vi "gds_simulator.vi"() -> ()   [LabVIEW 2012]
uses:
  <vilib>/addons/Modulation/Analog/controls/Complex Data Waveform.ctl
  <vilib>/addons/Modulation/niAMT.lvlib
panel:
  in  "RX Parameters":T1={"Sampling Rate"=4000000.0, "RX Oversample Factor"=4} {"Sampling Rate" format="%^.2e"}
  in  "Shared Parameters":T2={"Packet Length"=100, "Preamble Length"=20, "modulation type"=enum."OOK", "FSK deviation (Hz)"=150000.0, "Filter Parameters"={"modulation type"=enum."ASK", "pulse shaping filter (none)"=enum."none", "filter length (symbols)"=8, "filter parameter"=0.5}} {"Filter Parameters"."filter parameter" format="%.2f"; "FSK deviation (Hz)" format="%.2p"}
  out "Measurements":T3 caption="measurements" {"FSK error (Hz)" format="%.2f"; "deviation error (Hz)" format="%.2f"; "frequency drift (Hz)" format="%.2f"; "frequency offset (Hz)" format="%.2f"}
  out "recovered complex waveform":T4={"t0"=0.0, "dt"=6.25e-08, "Y"=[1.000128536665126+0.0i, 0.751586197118696+0.0i, 0.4998027919805991+0.0i, 0.250727982644391+0.0i, -0.00043487880682959964+0.0i, 0.2509497723379846+0.0i, 0.5004826812037222+0.0i, 0.7513401422859647+0.0i, 1.0011385612332764+0.0i, 0.7507480417630159+0.0i, 0.5005377871325838+0.0i, 0.2501383829137712+0.0i, 9.932713849573499e-05+0.0i, 0.2506331619076792+0.0i, 0.5007823017747152+0.0i, 0.7512111584953517+0.0i, 1.001234869577084+0.0i, 0.7507086660409406+0.0i, 0.5005559492379272+0.0i, 0.2501286476641118+0.0i, 0.00010432492947821529+0.0i, 0.2506307378836997+0.0i, 0.5007833967235412+0.0i, 0.7512107089735025+0.0i, 1.0012350317081362+0.0i, 0.7507086187539144+0.0i, 0.5005559599140732+0.0i, 0.2501286476641118+0.0i, 0.00010432492947821529+0.0i, 0.2506307378836997+0.0i, 0.5007833967235412+0.0i, 0.7512107089735025+0.0i, 1.0012350317081362+0.0i, 0.7507086187539144+0.0i, 0.5005559599140732+0.0i, 0.2501286476641118+0.0i, 0.00010432492947821529+0.0i, 0.2506307378836997+0.0i, 0.5007833967235412+0.0i, 0.7512107089735025+0.0i, 1.0012350317081362+0.0i, 0.7507086187539144+0.0i, 0.5005559599140732+0.0i, 0.2501286476641118+0.0i, 0.00010431423258635818+0.0i, 0.25063078524390886+0.0i, 0.5007832236720497+0.0i, 0.751211206406983+0.0i, 1.0012337838864194+0.0i, 0.7507114479511843+0.0i, 0.5005500450136401+0.0i, 0.25014027313937504+0.0i, 8.257686503592398e-05+0.0i, 0.2506699648285502+0.0i, 0.5007141646378572+0.0i, 0.7513334715067744+0.0i, 1.0009882953333455+0.0i, 0.751007662665835+0.0i, 0.5000017970341639+0.0i, 0.2506829533097328+0.0i, -0.0006056489582923521+0.0i, 0.2513390899485713+0.0i, 0.5002702293185063+0.0i, 0.7516085932252198+0.0i, 1.001317612226754+0.0i, 0.7502187599744155+0.0i, 0.5016154889194743+0.0i, 0.24853596070855516+0.0i, 0.0021738712548351516+0.0i, -0.0023391492054576648+0.0i, 0.002800740735483542+0.0i, -0.0025125144170003496+0.0i, 0.0025002679488030075+0.0i, 0.24875267224128303+0.0i, 0.502021464333328+0.0i, 0.7507211811248449+0.0i, 1.0011583479909132+0.0i, 1.00220487833868+0.0i, 0.9999033167533267+0.0i, 1.003155986548728+0.0i, 0.9991551723685784+0.0i, 1.0034766480326627+0.0i, 0.9989246775240931+0.0i, 1.0034343879039176+0.0i, 0.9990847189746185+0.0i, 1.0032604247248458+0.0i, 0.9994047431658972+0.0i, 1.002969462571593+0.0i, 0.9998314632099634+0.0i, 1.002477135847846+0.0i, 1.0003820743630871+0.0i, 1.0018633881693497+0.0i, 1.0009184881961803+0.0i, 0.7507665394691232+0.0i, 0.5006961121670002+0.0i, 0.24988702932257933+0.0i, 0.0003055397879960537+0.0i, 0.25045279064926845+0.0i, 0.5008598268147144+0.0i, 0.7512071510453188+0.0i, 1.0013382778946756+0.0i, 0.7505707278325852+0.0i, 0.5011013471120391+0.0i, 0.24929199517568223+0.0i, 0.0015231595958228514+0.0i, -0.0018697074439847532+0.0i, 0.0027112989756689007+0.0i, -0.0029122396150171115+0.0i, 0.0034003770436542204+0.0i, -0.003280540022698962+0.0i, 0.0032442710783317703+0.0i, -0.002660712780105675+0.0i, 0.0022979706937644286+0.0i, 0.2493218142787346+0.0i, 0.5013616603490355+0.0i, 0.7516035360534278+0.0i, 1.0001576644674623+0.0i, 1.0031112075731934+0.0i, 0.9987144979671289+0.0i, 1.004146722051281+0.0i, 0.9979277314279233+0.0i, 1.0046493566037573+0.0i, 0.9977125025638586+0.0i, 1.00456120393046+0.0i, 0.9981645620498365+0.0i, 1.0038346518801036+0.0i, 0.9993092785373742+0.0i, 1.0024797949898978+0.0i, 1.000977081790544+0.0i, 0.7501153376048973+0.0i, 0.5022282822062422+0.0i, 0.2477947265761407+0.0i, 0.003037807810337781+0.0i, -0.0031683564583393406+0.0i, 0.0033028481784962795+0.0i, -0.002764074700312304+0.0i, 0.0022269056021686183+0.0i, 0.24948848254532183+0.0i, 0.5008020006605832+0.0i, 0.7523023342756078+0.0i, 0.9992556274212987+0.0i, 1.004070814828902+0.0i, 0.9980292197466102+0.0i, 1.0045577684621514+0.0i, 0.9981298873906143+0.0i, 0.7531425834272562+0.0i, 0.498758723598838+0.0i, 0.25092847185712436+0.0i, -8.720643290498419e-05+0.0i, -0.0007035824731183089+0.0i, 0.0012974559681197394+0.0i, -0.0016541739776803268+0.0i, 0.0019144379726028931+0.0i, -0.0018236610274930329+0.0i, 0.0018481729222402153+0.0i, -0.0015247815861743777+0.0i, 0.0015178830543329+0.0i, -0.0011643152359881285+0.0i, 0.001333604266534931+0.0i, -0.0010725457022508302+0.0i, 0.0012734272337872686+0.0i, -0.0011993122929242345+0.0i, 0.001230254232285946+0.0i, -0.0011446387399175772+0.0i, 0.0009456776883348441+0.0i, -0.0006173716355468945+0.0i, 0.0001713033320193535+0.0i, 0.00035419013214571315+0.0i, -0.0008745850549463164+0.0i, 0.2520177269110101+0.0i, 0.49878953607777865+0.0i, 0.7533668501633469+0.0i, 0.9988846730300079+0.0i, 0.7528403690283272+0.0i, 0.4986174953520837+0.0i, 0.25141652289930166+0.0i, -0.0007302000338936521+0.0i, 1.8445209841694958e-05+0.0i, 0.0008521844813141006+0.0i, -0.001426765919450218+0.0i, 0.0021852452925184536+0.0i, -0.002528438837859647+0.0i, 0.002997879955148735+0.0i, -0.0029733308332217296+0.0i, 0.00315082717819+0.0i, -0.002686677203146186+0.0i, 0.0025721301595158634+0.0i, -0.0017725634728387057+0.0i, 0.0012947516375175863+0.0i, 0.25022918449120357+0.0i, 0.5001723228969468+0.0i, 0.7525948635635091+0.0i, 0.998928932959013+0.0i, 1.004286840061977+0.0i, 0.9974960620034783+0.0i, 1.0052861584200483+0.0i, 0.996983320098374+0.0i, 1.0052685164586146+0.0i, 0.997535802997294+0.0i, 1.0042180472660442+0.0i, 0.999018700305025+0.0i, 0.7518531806360466+0.0i, 0.5004569444288187+0.0i, 0.2492225895841184+0.0i, 0.0018712067029053039+0.0i, -0.0024738914890061643+0.0i, 0.003144292967198615+0.0i, -0.003227119370524421+0.0i, 0.0033750699927966995+0.0i, -0.0029067753001163275+0.0i, 0.0027240533397893457+0.0i, -0.0019115042765191893+0.0i, 0.001668999300507921+0.0i, 0.24974726959814494+0.0i, 0.5013532809643555+0.0i, 0.7510568970786982+0.0i, 1.0013505124478064+0.0i, 0.750694697032428+0.0i, 0.5006422807187524+0.0i, 0.24994025418320215+0.0i, 0.0003180831497285305+0.0i, 0.25037272173274683+0.0i, 0.5009492404030507+0.0i, 0.7512198666659388+0.0i, 1.0010681938167683+0.0i, 1.0018149964616638+0.0i, 1.0004066247126289+0.0i, 1.0024626621963892+0.0i, 0.9998401406350473+0.0i, 1.0029656343411324+0.0i, 0.9994027843429939+0.0i, 1.0032701050433652+0.0i, 0.9990626908536583+0.0i, 1.0034760306587285+0.0i, 0.9988505269792963+0.0i, 1.003607334783805+0.0i, 0.9988964615628683+0.0i, 1.003473011367319+0.0i, 0.999320307231625+0.0i, 1.0028137466748466+0.0i, 1.000289813496653+0.0i, 0.7509903364207922+0.0i, 0.5012302976192266+0.0i, 0.2487169225826871+0.0i, 0.002410405623408453+0.0i, -0.00291987165725027+0.0i, 0.003779971804916688+0.0i, -0.0038268655079649184+0.0i, 0.004110535871290194+0.0i, -0.003630565357746327+0.0i, 0.003249390516118569+0.0i, -0.002323934836355721+0.0i, 0.0016094346023591741+0.0i, 0.25019740462392726+0.0i, 0.5003631568518416+0.0i, 0.7525267742139664+0.0i, 0.9995277131733875+0.0i, 1.0033655402096595+0.0i, 0.9991790995867168+0.0i, 1.003109171928079+0.0i, 0.9997628421906146+0.0i, 0.7516202214600886+0.0i, 0.49999724949181384+0.0i, 0.2502284540865264+0.0i, -6.589272606641215e-05+0.0i, 0.25072496167122876+0.0i, 0.5002393515812941+0.0i, 0.7520858257592368+0.0i, 0.999896445421567+0.0i, 1.0030833798673002+0.0i, 0.9991670166932658+0.0i, 1.0034188121769922+0.0i, 0.9993540508400994+0.0i, 0.7521256538962483+0.0i, 0.5000108121518518+0.0i, 0.24990091650022914+0.0i, 0.0011619766526191919+0.0i, -0.001890333330762509+0.0i, 0.0025216283810360314+0.0i, -0.0027963893182235034+0.0i, 0.0028600957266303587+0.0i, -0.002443365051434658+0.0i, 0.0020252183474949803+0.0i, -0.0011821696422666657+0.0i, 0.0006650353876859234+0.0i, 0.25081418473018074+0.0i, 0.5001923724300027+0.0i, 0.7521715419278338+0.0i, 1.000404836638586+0.0i, 0.7513420128234725+0.0i, 0.5004019124642737+0.0i, 0.24971757851375342+0.0i, 0.0009254515422090878+0.0i, -0.0013072784905761145+0.0i, 0.0015366552183685134+0.0i, -0.0014704600390226075+0.0i, 0.0012280797189567999+0.0i, 0.24997914685265876+0.0i, 0.5007278870275318+0.0i, 0.7519862062856911+0.0i, 0.9999659431859507+0.0i, 1.003123626274542+0.0i, 0.9991721084481632+0.0i, 1.0033676802504412+0.0i, 0.9992980675412391+0.0i, 0.752206405410947+0.0i, 0.4995530880585731+0.0i, 0.2505871896585888+0.0i, 3.840712565549651e-05+0.0i, 0.2502234877139924+0.0i, 0.5013047898431594+0.0i, 0.7504903125448779+0.0i, 1.0019672595444384+0.0i, 0.7501129012488448+0.0i, 0.5011848796153869+0.0i, 0.24969454663249652+0.0i, 0.0006218040972395145+0.0i, 0.25016400162887775+0.0i, 0.5014883194234692+0.0i, 0.7504697015769647+0.0i, 1.0022607543615492+0.0i, 0.749602476677032+0.0i, 0.5017861005341123+0.0i, 0.24889124028170884+0.0i, 0.0012967371134894872+0.0i, 0.24968437818072936+0.0i, 0.5015779278579268+0.0i, 0.7508790789973246+0.0i, 1.001337647900318+0.0i, 1.0016802195521612+0.0i, 1.0004818855552846+0.0i, 1.0024205926838794+0.0i, 0.9998631170272833+0.0i, 1.0029535697147287+0.0i, 0.9994086933551652+0.0i, 1.0032677289310172+0.0i, 0.9990626787180361+0.0i, 1.0034784577675415+0.0i, 0.9988444387830785+0.0i, 1.003619907839004+0.0i, 0.9988722178342461+0.0i, 1.0035179440669189+0.0i, 0.9992390722935826+0.0i, 1.0029602575921268+0.0i, 0.9999983117774736+0.0i, 0.7513707581400929+0.0i, 0.5005314095645278+0.0i, 0.24952937363706787+0.0i, 0.0011826724906098807+0.0i, -0.0015683569883093978+0.0i, 0.0020767245475469733+0.0i, -0.0021723667472836323+0.0i, 0.002477891339365218+0.0i, -0.002314668615754756+0.0i, 0.002565432800982565+0.0i, -0.002272033507855293+0.0i, 0.002547378386111064+0.0i, -0.00227432748809499+0.0i, 0.0025701784528972074+0.0i, -0.0023221705674448213+0.0i, 0.002488878050033193+0.0i, -0.0021878228584384517+0.0i, 0.002100278455769505+0.0i, -0.0016116515915972904+0.0i, 0.0013193060538595086+0.0i, 0.25001015783076647+0.0i, 0.5007329728941675+0.0i, 0.7519443237220552+0.0i, 0.9998881996870254+0.0i, 1.0032460318429037+0.0i, 0.9986390640729825+0.0i, 1.0041892889972714+0.0i, 0.9979034965170791+0.0i, 1.0046642977876403+0.0i, 0.9977005055997629+0.0i, 1.004575702951552+0.0i, 0.998141556905516+0.0i, 1.0038743756338298+0.0i, 0.999239873644491+0.0i, 1.002602604810197+0.0i, 1.0007303347396035+0.0i, 0.7504143815168087+0.0i, 0.5016741193263274+0.0i, 0.2483490322217527+0.0i, 0.002327844619456096+0.0i, -0.0024600517536761735+0.0i, 0.0027898538249527204+0.0i, -0.002366687882076294+0.0i, 0.0023107446393984704+0.0i, 0.24899574720835296+0.0i, 0.5018676176179138+0.0i, 0.7506975244113171+0.0i, 1.0013482017234923+0.0i, 0.7510587295169913+0.0i, 0.5001222298991419+0.0i, 0.2506986647626669+0.0i, -0.0003326270705530104+0.0i, 0.2508397837456261+0.0i, 0.5008657137879676+0.0i, 0.7508080658462138+0.0i, 1.0019913095154176+0.0i, 0.7497396333351374+0.0i, 0.5017049245467311+0.0i, 0.24894538541593653+0.0i, 0.001250754117456808+0.0i, 0.2497385936696718+0.0i, 0.5014965257566558+0.0i, 0.7510168379851694+0.0i, 1.001066647862598+0.0i, 1.0020218637752867+0.0i, 0.9998522298305689+0.0i, 1.0031098310585427+0.0i, 0.9988833788086331+0.0i, 1.0040031165540595+0.0i, 0.9982658699811213+0.0i, 1.004355301703853+0.0i, 0.9981642624786498+0.0i, 1.0040410697450617+0.0i, 0.9987548834110189+0.0i, 1.0031274139985074+0.0i, 1.0000190828185553+0.0i, 0.7511556490150857+0.0i, 0.5010854529439307+0.0i, 0.24889154871188202+0.0i]} {"Y" format="%.3f"; "dt" format="%^.2e"; "t0" format="%.4f"}
  out "Transmitted Signal":T4={"t0"=0.0, "dt"=6.25e-08, "Y"=[1.0+0.0i, 1.0+0.0i, 0.0+0.0i, 0.0+0.0i, 0.0+0.0i, 0.0+0.0i, 1.0+0.0i, 1.0+0.0i, 1.0+0.0i, 1.0+0.0i, 0.0+0.0i, 0.0+0.0i, 0.0+0.0i, 0.0+0.0i, 1.0+0.0i, 1.0+0.0i, 1.0+0.0i, 1.0+0.0i, 0.0+0.0i, 0.0+0.0i, 0.0+0.0i, 0.0+0.0i, 1.0+0.0i, 1.0+0.0i, 1.0+0.0i, 1.0+0.0i, 0.0+0.0i, 0.0+0.0i, 0.0+0.0i, 0.0+0.0i, 1.0+0.0i, 1.0+0.0i, 1.0+0.0i, 1.0+0.0i, 0.0+0.0i, 0.0+0.0i, 0.0+0.0i, 0.0+0.0i, 1.0+0.0i, 1.0+0.0i, 1.0+0.0i, 1.0+0.0i, 0.0+0.0i, 0.0+0.0i, 0.0+0.0i, 0.0+0.0i, 1.0+0.0i, 1.0+0.0i, 1.0+0.0i, 1.0+0.0i, 0.0+0.0i, 0.0+0.0i, 0.0+0.0i, 0.0+0.0i, 1.0+0.0i, 1.0+0.0i, 1.0+0.0i, 1.0+0.0i, 0.0+0.0i, 0.0+0.0i, 0.0+0.0i, 0.0+0.0i, 1.0+0.0i, 1.0+0.0i, 1.0+0.0i, 1.0+0.0i, 0.0+0.0i, 0.0+0.0i, 0.0+0.0i, 0.0+0.0i, 1.0+0.0i, 1.0+0.0i, 1.0+0.0i, 1.0+0.0i, 0.0+0.0i, 0.0+0.0i, 0.0+0.0i, 0.0+0.0i, 1.0+0.0i, 1.0+0.0i, 1.0+0.0i, 1.0+0.0i, 0.0+0.0i, 0.0+0.0i, 0.0+0.0i, 0.0+0.0i, 1.0+0.0i, 1.0+0.0i, 1.0+0.0i, 1.0+0.0i, 0.0+0.0i, 0.0+0.0i, 0.0+0.0i, 0.0+0.0i, 0.0+0.0i, 0.0+0.0i, 0.0+0.0i, 0.0+0.0i, 0.0+0.0i, 0.0+0.0i, 0.0+0.0i, 0.0+0.0i, 1.0+0.0i, 1.0+0.0i, 1.0+0.0i, 1.0+0.0i, 0.0+0.0i, 0.0+0.0i, 0.0+0.0i, 0.0+0.0i, 0.0+0.0i, 0.0+0.0i, 0.0+0.0i, 0.0+0.0i, 1.0+0.0i, 1.0+0.0i, 1.0+0.0i, 1.0+0.0i, 0.0+0.0i, 0.0+0.0i, 0.0+0.0i, 0.0+0.0i, 0.0+0.0i, 0.0+0.0i, 0.0+0.0i, 0.0+0.0i, 1.0+0.0i, 1.0+0.0i, 1.0+0.0i, 1.0+0.0i, 0.0+0.0i, 0.0+0.0i, 0.0+0.0i, 0.0+0.0i, 0.0+0.0i, 0.0+0.0i, 0.0+0.0i, 0.0+0.0i, 0.0+0.0i, 0.0+0.0i, 0.0+0.0i, 0.0+0.0i, 1.0+0.0i, 1.0+0.0i, 1.0+0.0i, 1.0+0.0i, 1.0+0.0i, 1.0+0.0i, 1.0+0.0i, 1.0+0.0i, 1.0+0.0i, 1.0+0.0i, 1.0+0.0i, 1.0+0.0i, 0.0+0.0i, 0.0+0.0i, 0.0+0.0i, 0.0+0.0i, 1.0+0.0i, 1.0+0.0i, 1.0+0.0i, 1.0+0.0i, 0.0+0.0i, 0.0+0.0i, 0.0+0.0i, 0.0+0.0i, 0.0+0.0i, 0.0+0.0i, 0.0+0.0i, 0.0+0.0i, 1.0+0.0i, 1.0+0.0i, 1.0+0.0i, 1.0+0.0i, 1.0+0.0i, 1.0+0.0i, 1.0+0.0i, 1.0+0.0i, 1.0+0.0i, 1.0+0.0i, 1.0+0.0i, 1.0+0.0i, 0.0+0.0i, 0.0+0.0i, 0.0+0.0i, 0.0+0.0i, 1.0+0.0i, 1.0+0.0i, 1.0+0.0i, 1.0+0.0i, 0.0+0.0i, 0.0+0.0i, 0.0+0.0i, 0.0+0.0i, 0.0+0.0i, 0.0+0.0i, 0.0+0.0i, 0.0+0.0i, 0.0+0.0i, 0.0+0.0i, 0.0+0.0i, 0.0+0.0i, 1.0+0.0i, 1.0+0.0i, 1.0+0.0i, 1.0+0.0i, 0.0+0.0i, 0.0+0.0i, 0.0+0.0i, 0.0+0.0i, 1.0+0.0i, 1.0+0.0i, 1.0+0.0i, 1.0+0.0i, 0.0+0.0i, 0.0+0.0i, 0.0+0.0i, 0.0+0.0i, 1.0+0.0i, 1.0+0.0i, 1.0+0.0i, 1.0+0.0i, 0.0+0.0i, 0.0+0.0i, 0.0+0.0i, 0.0+0.0i, 0.0+0.0i, 0.0+0.0i, 0.0+0.0i, 0.0+0.0i, 0.0+0.0i, 0.0+0.0i, 0.0+0.0i, 0.0+0.0i, 0.0+0.0i, 0.0+0.0i, 0.0+0.0i, 0.0+0.0i, 1.0+0.0i, 1.0+0.0i, 1.0+0.0i, 1.0+0.0i, 0.0+0.0i, 0.0+0.0i, 0.0+0.0i, 0.0+0.0i, 1.0+0.0i, 1.0+0.0i, 1.0+0.0i, 1.0+0.0i, 0.0+0.0i, 0.0+0.0i, 0.0+0.0i, 0.0+0.0i, 1.0+0.0i, 1.0+0.0i, 1.0+0.0i, 1.0+0.0i, 0.0+0.0i, 0.0+0.0i, 0.0+0.0i, 0.0+0.0i, 1.0+0.0i, 1.0+0.0i, 1.0+0.0i, 1.0+0.0i, 0.0+0.0i, 0.0+0.0i, 0.0+0.0i, 0.0+0.0i, 1.0+0.0i, 1.0+0.0i, 1.0+0.0i, 1.0+0.0i, 0.0+0.0i, 0.0+0.0i, 0.0+0.0i, 0.0+0.0i, 1.0+0.0i, 1.0+0.0i, 1.0+0.0i, 1.0+0.0i, 0.0+0.0i, 0.0+0.0i, 0.0+0.0i, 0.0+0.0i, 1.0+0.0i, 1.0+0.0i, 1.0+0.0i, 1.0+0.0i, 0.0+0.0i, 0.0+0.0i, 0.0+0.0i, 0.0+0.0i, 1.0+0.0i, 1.0+0.0i, 1.0+0.0i, 1.0+0.0i, 0.0+0.0i, 0.0+0.0i, 0.0+0.0i, 0.0+0.0i, 1.0+0.0i, 1.0+0.0i, 1.0+0.0i, 1.0+0.0i, 1.0+0.0i, 1.0+0.0i, 1.0+0.0i, 1.0+0.0i, 0.0+0.0i, 0.0+0.0i, 0.0+0.0i, 0.0+0.0i, 1.0+0.0i, 1.0+0.0i, 1.0+0.0i, 1.0+0.0i, 0.0+0.0i, 0.0+0.0i, 0.0+0.0i, 0.0+0.0i, 0.0+0.0i, 0.0+0.0i, 0.0+0.0i, 0.0+0.0i, 0.0+0.0i, 0.0+0.0i, 0.0+0.0i, 0.0+0.0i, 1.0+0.0i, 1.0+0.0i, 1.0+0.0i, 1.0+0.0i, 1.0+0.0i, 1.0+0.0i, 1.0+0.0i, 1.0+0.0i, 0.0+0.0i, 0.0+0.0i, 0.0+0.0i, 0.0+0.0i, 1.0+0.0i, 1.0+0.0i, 1.0+0.0i, 1.0+0.0i, 0.0+0.0i, 0.0+0.0i, 0.0+0.0i, 0.0+0.0i, 0.0+0.0i, 0.0+0.0i, 0.0+0.0i, 0.0+0.0i, 0.0+0.0i, 0.0+0.0i, 0.0+0.0i, 0.0+0.0i, 1.0+0.0i, 1.0+0.0i, 1.0+0.0i, 1.0+0.0i, 1.0+0.0i, 1.0+0.0i, 1.0+0.0i, 1.0+0.0i, 0.0+0.0i, 0.0+0.0i, 0.0+0.0i, 0.0+0.0i, 0.0+0.0i, 0.0+0.0i, 0.0+0.0i, 0.0+0.0i, 1.0+0.0i, 1.0+0.0i, 1.0+0.0i, 1.0+0.0i, 1.0+0.0i, 1.0+0.0i, 1.0+0.0i, 1.0+0.0i, 1.0+0.0i, 1.0+0.0i, 1.0+0.0i, 1.0+0.0i, 0.0+0.0i, 0.0+0.0i, 0.0+0.0i, 0.0+0.0i, 0.0+0.0i, 0.0+0.0i, 0.0+0.0i, 0.0+0.0i, 0.0+0.0i, 0.0+0.0i, 0.0+0.0i, 0.0+0.0i, 1.0+0.0i, 1.0+0.0i, 1.0+0.0i, 1.0+0.0i, 0.0+0.0i, 0.0+0.0i, 0.0+0.0i, 0.0+0.0i, 1.0+0.0i, 1.0+0.0i, 1.0+0.0i, 1.0+0.0i, 1.0+0.0i, 1.0+0.0i, 1.0+0.0i, 1.0+0.0i, 1.0+0.0i, 1.0+0.0i, 1.0+0.0i, 1.0+0.0i, 0.0+0.0i, 0.0+0.0i, 0.0+0.0i, 0.0+0.0i, 0.0+0.0i, 0.0+0.0i, 0.0+0.0i, 0.0+0.0i, 1.0+0.0i, 1.0+0.0i, 1.0+0.0i, 1.0+0.0i, 1.0+0.0i, 1.0+0.0i, 1.0+0.0i, 1.0+0.0i, 1.0+0.0i, 1.0+0.0i, 1.0+0.0i, 1.0+0.0i, 0.0+0.0i, 0.0+0.0i, 0.0+0.0i, 0.0+0.0i, 0.0+0.0i, 0.0+0.0i, 0.0+0.0i, 0.0+0.0i, 1.0+0.0i, 1.0+0.0i, 1.0+0.0i, 1.0+0.0i, 0.0+0.0i, 0.0+0.0i, 0.0+0.0i, 0.0+0.0i, 1.0+0.0i, 1.0+0.0i, 1.0+0.0i, 1.0+0.0i, 0.0+0.0i, 0.0+0.0i, 0.0+0.0i, 0.0+0.0i, 1.0+0.0i, 1.0+0.0i, 1.0+0.0i, 1.0+0.0i, 1.0+0.0i, 1.0+0.0i, 1.0+0.0i, 1.0+0.0i, 1.0+0.0i, 1.0+0.0i, 1.0+0.0i, 1.0+0.0i, 1.0+0.0i, 1.0+0.0i, 1.0+0.0i, 1.0+0.0i]} {"Y" format="%.3f"; "dt" format="%^.2e"; "t0" format="%.4f"}
  out "symbols out":cdb[](array[numeric])=[1.0+0.0i, 0.0+0.0i, 1.0+0.0i, 0.0+0.0i, 1.0+0.0i, 0.0+0.0i, 1.0+0.0i, 0.0+0.0i, 1.0+0.0i, 0.0+0.0i, 1.0+0.0i, 0.0+0.0i, 1.0+0.0i, 0.0+0.0i, 1.0+0.0i, 0.0+0.0i, 1.0+0.0i, 0.0+0.0i, 1.0+0.0i, 0.0+0.0i, 0.0+0.0i, 1.0+0.0i, 0.0+0.0i, 0.0+0.0i, 0.0+0.0i, 0.0+0.0i, 1.0+0.0i, 0.0+0.0i, 0.0+0.0i, 0.0+0.0i, 1.0+0.0i, 0.0+0.0i, 1.0+0.0i, 1.0+0.0i, 1.0+0.0i, 0.0+0.0i, 0.0+0.0i, 1.0+0.0i, 1.0+0.0i, 0.0+0.0i, 1.0+0.0i, 0.0+0.0i, 0.0+0.0i, 0.0+0.0i, 1.0+0.0i, 1.0+0.0i, 0.0+0.0i, 1.0+0.0i, 1.0+0.0i, 0.0+0.0i, 1.0+0.0i, 0.0+0.0i, 0.0+0.0i, 1.0+0.0i, 1.0+0.0i, 1.0+0.0i, 0.0+0.0i, 1.0+0.0i, 1.0+0.0i, 1.0+0.0i, 1.0+0.0i, 1.0+0.0i, 1.0+0.0i, 0.0+0.0i, 1.0+0.0i, 0.0+0.0i, 1.0+0.0i, 0.0+0.0i, 0.0+0.0i, 1.0+0.0i, 0.0+0.0i, 1.0+0.0i, 1.0+0.0i, 1.0+0.0i, 1.0+0.0i, 0.0+0.0i, 0.0+0.0i, 0.0+0.0i, 1.0+0.0i, 1.0+0.0i, 0.0+0.0i, 0.0+0.0i, 0.0+0.0i, 1.0+0.0i, 0.0+0.0i, 0.0+0.0i, 1.0+0.0i, 1.0+0.0i, 1.0+0.0i, 0.0+0.0i, 0.0+0.0i, 0.0+0.0i, 0.0+0.0i, 1.0+0.0i, 1.0+0.0i, 1.0+0.0i, 0.0+0.0i, 0.0+0.0i, 1.0+0.0i, 1.0+0.0i, 1.0+0.0i, 1.0+0.0i, 1.0+0.0i, 0.0+0.0i, 0.0+0.0i, 0.0+0.0i, 0.0+0.0i, 1.0+0.0i, 1.0+0.0i, 0.0+0.0i, 0.0+0.0i, 1.0+0.0i, 0.0+0.0i, 1.0+0.0i, 0.0+0.0i, 0.0+0.0i, 1.0+0.0i, 0.0+0.0i, 1.0+0.0i, 1.0+0.0i] caption="Modulated Symbols" format="%.2f"
  in  "TX Parameters":T5={"Sampling Rate"=4000000.0, "Oversample Factor"=4} {"Sampling Rate" format="%^.2e"}
  out "BER":dbl=-1.0
  out "Recovered Bit Sequence":i8[](array[numeric])
  out "error out":errorcluster
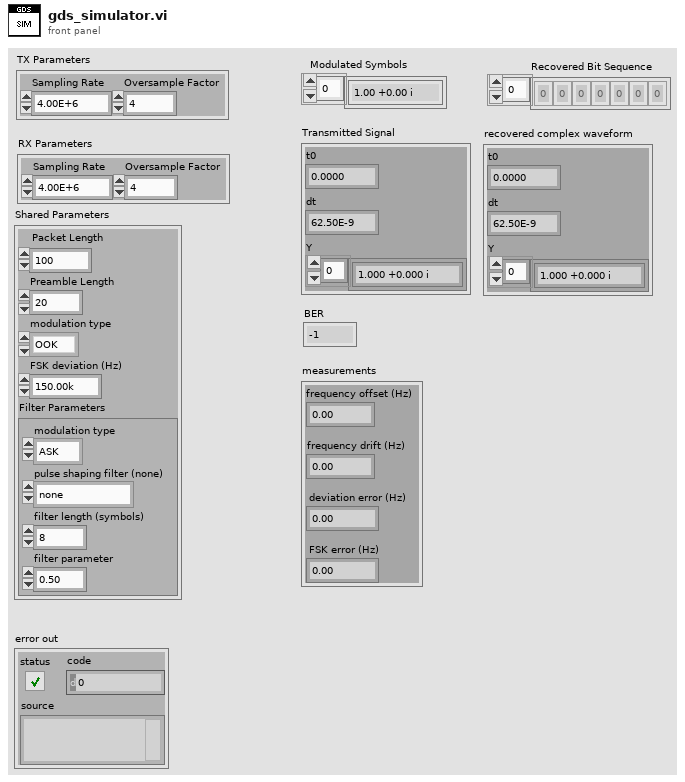
[diagram p1: front panel]
types:
  T1 = cluster{"Sampling Rate":dbl, "RX Oversample Factor":i32}
  T2 = cluster{"Packet Length":i32, "Preamble Length":i32, "modulation type":enum16{"OOK", "FSK", "PSK", "QAM", "MSK", "PAM", "ASK", "CPM"}, "FSK deviation (Hz)":dbl, "Filter Parameters":cluster{"modulation type":enum16{"FSK", "PSK", "QAM", "MSK", "PAM", "ASK", "CPM"}, "pulse shaping filter (none)":enum16{"none", "Raised Cosine", "Root Raised Cos", "Gaussian"}, "filter length (symbols)":i32, "filter parameter":dbl}}
  T3 = cluster{"frequency offset (Hz)":dbl, "frequency drift (Hz)":dbl, "deviation error (Hz)":dbl, "FSK error (Hz)":dbl}
  T4 = typedef "niAMT.lvlib/Complex Data Waveform.ctl" = cluster{"t0":dbl, "dt":dbl, "Y":cdb[]}
  T5 = cluster{"Sampling Rate":dbl, "Oversample Factor":i32}
  T6 = cluster{"TX Parameters":cluster{"Sampling Rate":dbl, "Oversample Factor":i32}, "Shared Parameters":cluster{"Packet Length":i32, "Preamble Length":i32, "modulation type":enum16{"OOK", "FSK", "PSK", "QAM", "MSK", "PAM", "ASK", "CPM"}, "FSK deviation (Hz)":dbl, "Filter Parameters":cluster{"modulation type":enum16{"FSK", "PSK", "QAM", "MSK", "PAM", "ASK", "CPM"}, "pulse shaping filter (none)":enum16{"none", "Raised Cosine", "Root Raised Cos", "Gaussian"}, "filter length (symbols)":i32, "filter parameter":dbl}}}
  T7 = cluster{"RX Parameters":cluster{"Sampling Rate":dbl, "RX Oversample Factor":i32}, "Shared Parameters":cluster{"Packet Length":i32, "Preamble Length":i32, "modulation type":enum16{"OOK", "FSK", "PSK", "QAM", "MSK", "PAM", "ASK", "CPM"}, "FSK deviation (Hz)":dbl, "Filter Parameters":cluster{"modulation type":enum16{"FSK", "PSK", "QAM", "MSK", "PAM", "ASK", "CPM"}, "pulse shaping filter (none)":enum16{"none", "Raised Cosine", "Root Raised Cos", "Gaussian"}, "filter length (symbols)":i32, "filter parameter":dbl}}}
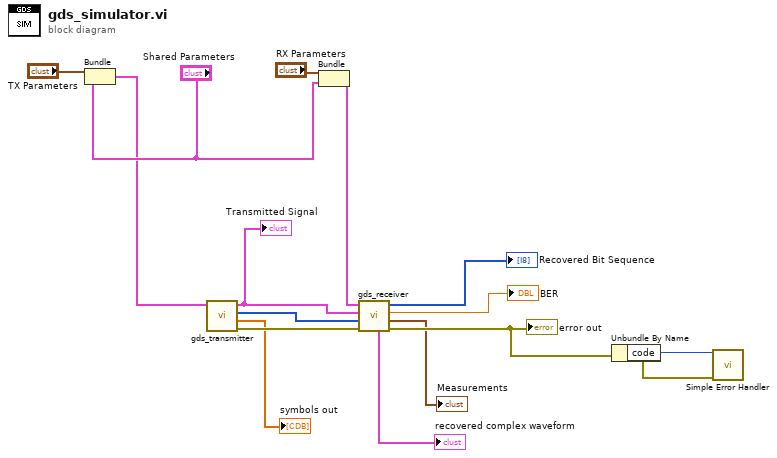
[diagram p0: block diagram]
diagram:
  n1 = Bundle("TX Parameters"="TX Parameters", "Shared Parameters"="Shared Parameters") -> (w5:T6)  [unwired: 1 in]
  n2 = call "gds_transmitter.vi"("Modulation Parameters"=w5) -> ("error out"=w15:errorcluster, "Symbols Out"=→"symbols out":cdb[], "Key Bit Sequence"=w3:i8[], "Transmitted Signal"=w4:T4)  [unwired: 7 in]
  "Transmitted Signal" <- w4
  n3 = Bundle("RX Parameters"="RX Parameters", "Shared Parameters"="Shared Parameters") -> (w2:T7)  [unwired: 1 in]
  n4 = call "gds_receiver.vi"("error in (no error)"=w15, "Received Bit Sequence"=w3, "Received Signal"=w4, "Modulation Parameters"=w2) -> ("error out"=w10:errorcluster, "Measurements"=→"Measurements":T3, "BER"=→"BER":dbl, "Key Bit Sequence"=→"Recovered Bit Sequence":i8[], "recovered complex waveform"=→"recovered complex waveform":T4)  [unwired: 3 in]
  "error out" <- w10
  n5 = Unbundle By Name(w10) -> ("code"=w11:i32)
  n6 = call <vilib>:"Simple Error Handler.vi"("error code (no error:0)"=w11, "error in (no error)"=w10) -> ()  [unwired: 3 in, 5 out]
